vi "GetCoreVersion.vi"(5 "error in (no error)":errorcluster) -> (15 "GetAvailableBrowserVersionString":string, 19 "error out":errorcluster)   [LabVIEW 2020, in "DP_WebView.lvclass"]
uses:
  DP_WebView.lvclass
  C:/Projects/DependencyViewer/DependencyViewer/DP_WebView_class/data/Microsoft.Web.WebView2.Core.dll
  data/Microsoft.Web.WebView2.Core.dll
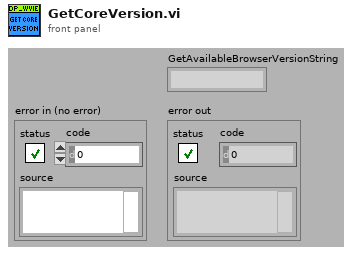
[diagram p1: front panel]
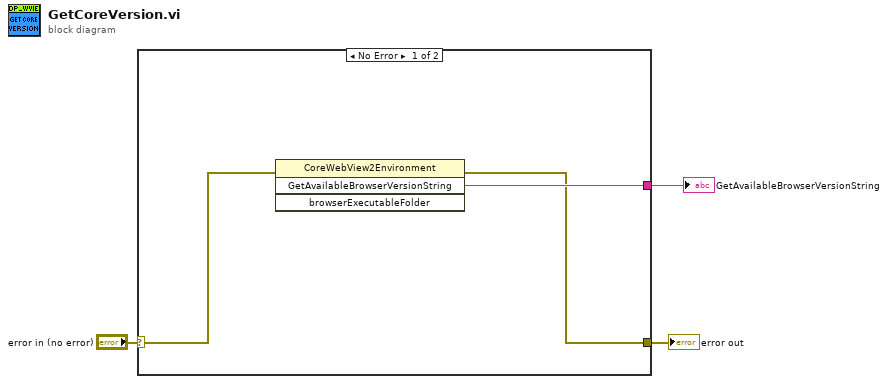
[diagram p0: block diagram]
diagram:
  n1 = case shown="No Error" "error in (no error)" {
    selector: "error in (no error)" -> [w5 w7]
    tunnel: [w4 w7] -> w2
    tunnel: [w6 _] -> w1
    frame No Error {
      n2 = invoke class="CoreWebView2Environment" method="GetAvailableBrowserVersionString"(error in=w5) -> (error out=w4:errorcluster, "GetAvailableBrowserVersionString"=w6:string)  [unwired: 3 in, 2 out]
    }
    frame Error {
    }
  }
  "error out" <- w2
  "GetAvailableBrowserVersionString" <- w1
